vi "Create Frame (empty).vi"(6 "stylename":string, 8 "error in (no error)":errorcluster, 11 "ooWriter in":refnum<class "ooWriter.lvclass">) -> (0 "error out":errorcluster, 2 "Frame (graphic)":refnum<k24>, 3 "ooWriter out":refnum<class "ooWriter.lvclass">)   [LabVIEW 2009, in "ooWriter.lvclass"]
uses:
  ooWriter.lvclass
  C:/Projets/LAVAG/OpenOfficeRGT/AODL/DLLs/AODL.dll
  ooWriter.lvclass/ooWriter.ctl
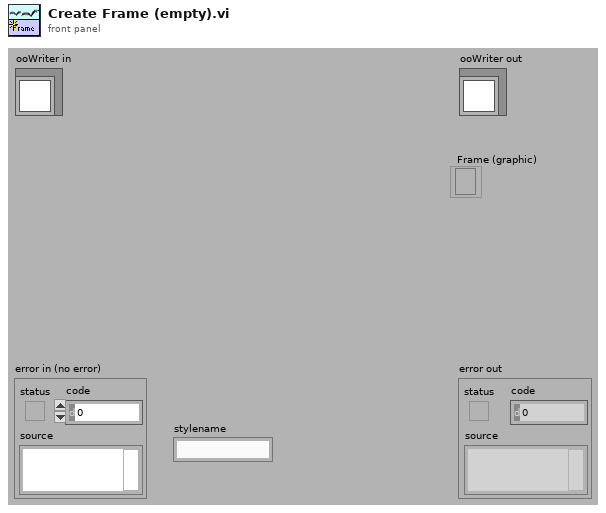
[diagram p1: front panel]
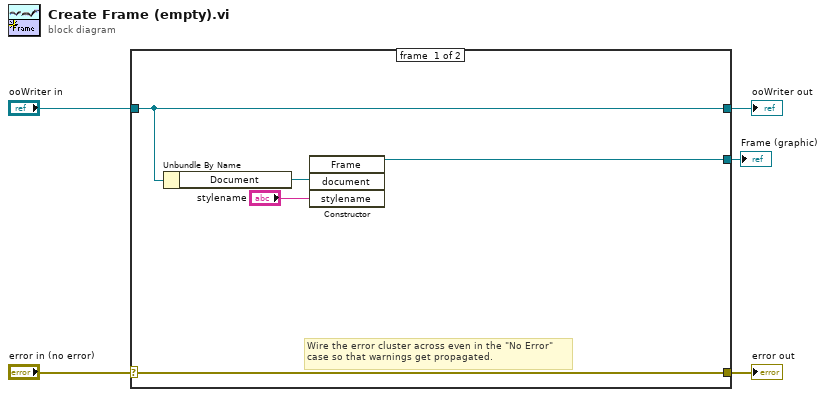
[diagram p0: block diagram]
diagram:
  n1 = case shown="No Error" "error in (no error)" {
    selector: "error in (no error)" -> [w10 w12]
    tunnel: [w10 w12] -> w4
    tunnel: [w9 w11] -> w2
    tunnel: "ooWriter in" -> [w9 w11]
    tunnel: [w6 _] -> w1
    frame #0 {
      # "Wire the error cluster across even in the \"No Error\"\ncase so that warnings get propagated."
      n2 = Unbundle By Name(w9) -> ("Document"=w8:refnum<k24>)
      n3 = constructor class="Frame"("document"=w8, "stylename"="stylename") -> (reference out=w6:refnum<k24>)  [unwired: 3 in, 4 out]
    }
    frame #1 {
    }
  }
  "error out" <- w4
  "ooWriter out" <- w2
  "Frame (graphic)" <- w1
